vi "Simple Math.vi"() -> ()   [LabVIEW 2010]
panel:
  out "X * Y =":i16
  out "X - Y =":i16
  out "X + Y =":i16
  in  "Y":i16
  in  "X":i16
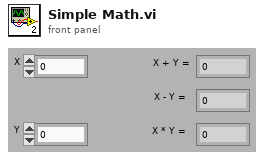
[diagram p1: front panel]
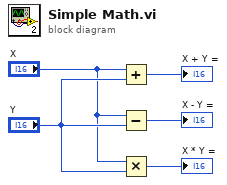
[diagram p0: block diagram]
diagram:
  n1 = Add(x="X", y="Y") -> (x+y=→"X + Y =":i16)
  n2 = Subtract(x="X", y="Y") -> (x-y=→"X - Y =":i16)
  n3 = Multiply(x="X", y="Y") -> (x*y=→"X * Y =":i16)
